vi "Init Airmar Serial.vi"(8 "error in (no error)":errorcluster, 10 "NotifierReff":T1, 11 "VISA Refnum in":refnum<visa-resource-name>="COM1") -> (0 "error out":errorcluster, 2 "Total number of connection attempts":i32, 3 "VISA Refnum out":refnum<visa-resource-name>)   [LabVIEW 2013]
doc: "This VI checks to see if the sensor is communicating on 4800 or 38400 baud and sets it to 38400 baud if it is not already."
uses:
  Data/TypeDefs/UTM Location.ctl
  Data/TypeDefs/Sail Set Suggestions.ctl
  Data/TypeDefs/Rudder Set Suggestions.ctl
  Data/TypeDefs/Notifiers.ctl
  Data/TypeDefs/OverrideMode.ctl
  Data/TypeDefs/OverrideInformation.ctl
  Data/TypeDefs/DynamixelSetupInfo.ctl
  Data/TypeDefs/MotorSetup.ctl
  Data/TypeDefs/AirmarStatus.ctl
panel:
  out "# of 38400 baud attempts":i32
  out "# of 4800 baud attempts":i32
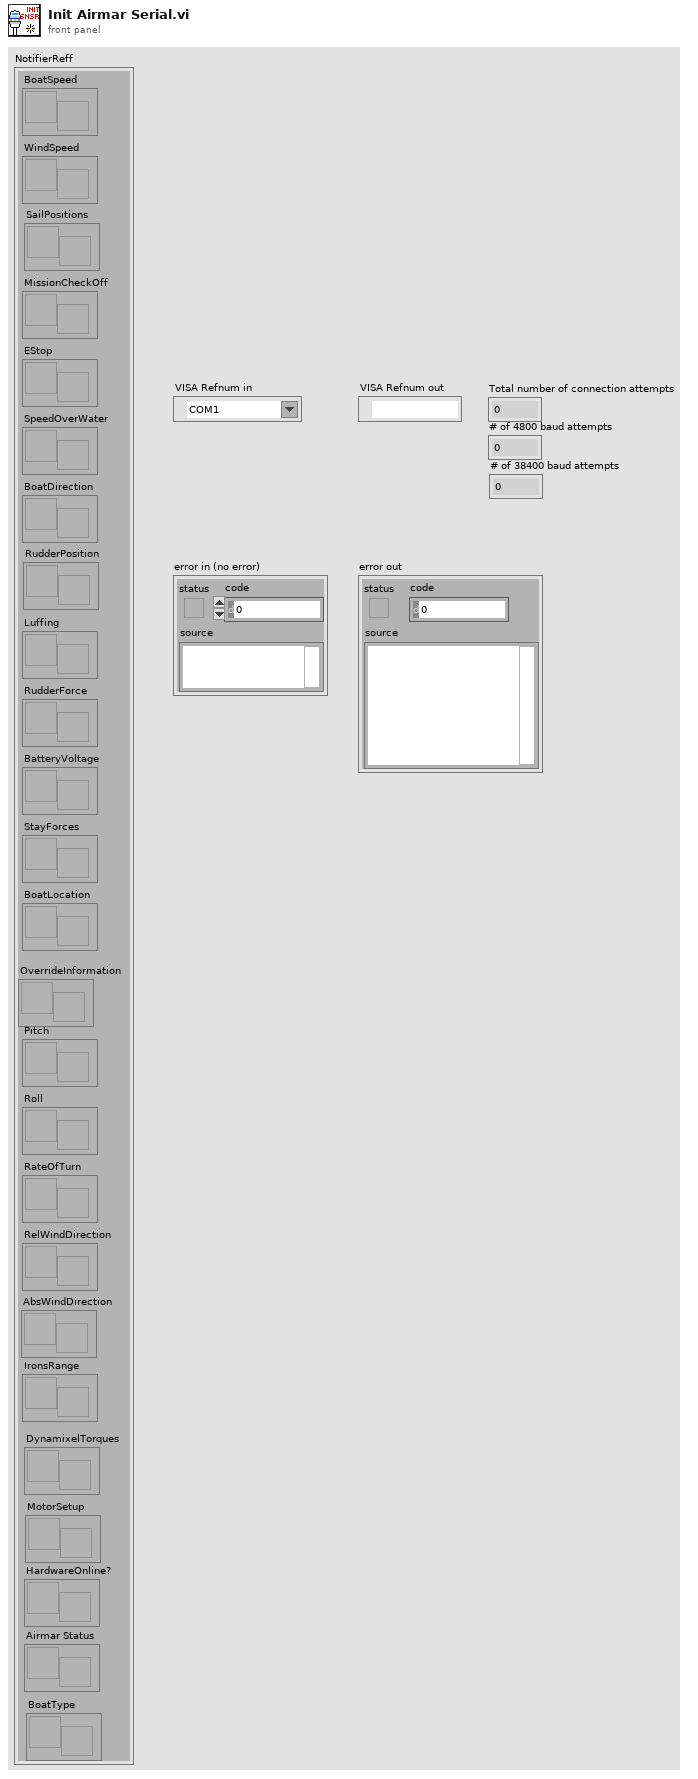
[diagram p1: front panel]
types:
  T1 = typedef "Notifiers.ctl" = cluster{"BoatSpeed":refnum<notifier>, "WindSpeed":refnum<notifier>, "MissionCheckOff":refnum<notifier>, "EStop":refnum<notifier>, "SpeedOverWater":refnum<notifier>, "BoatDirection":refnum<notifier>, "Luffing":refnum<notifier>, "RudderForce":refnum<notifier>, "BatteryVoltage":refnum<notifier>, "StayForces":refnum<notifier>, "BoatLocation":refnum<notifier>, "Pitch":refnum<notifier>, "Roll":refnum<notifier>, "RateOfTurn":refnum<notifier>, "RelWindDirection":refnum<notifier>, "SailPositions":refnum<notifier>, "RudderPosition":refnum<notifier>, "IronsRange":refnum<notifier>, "AbsWindDirection":refnum<notifier>, "OverrideInformation":refnum<notifier>, "DynamixelTorques":refnum<notifier>, "HardwareOnline?":refnum<notifier>, "MotorSetup":refnum<notifier>, "Airmar Status":refnum<notifier>, "BoatType":refnum<notifier>}
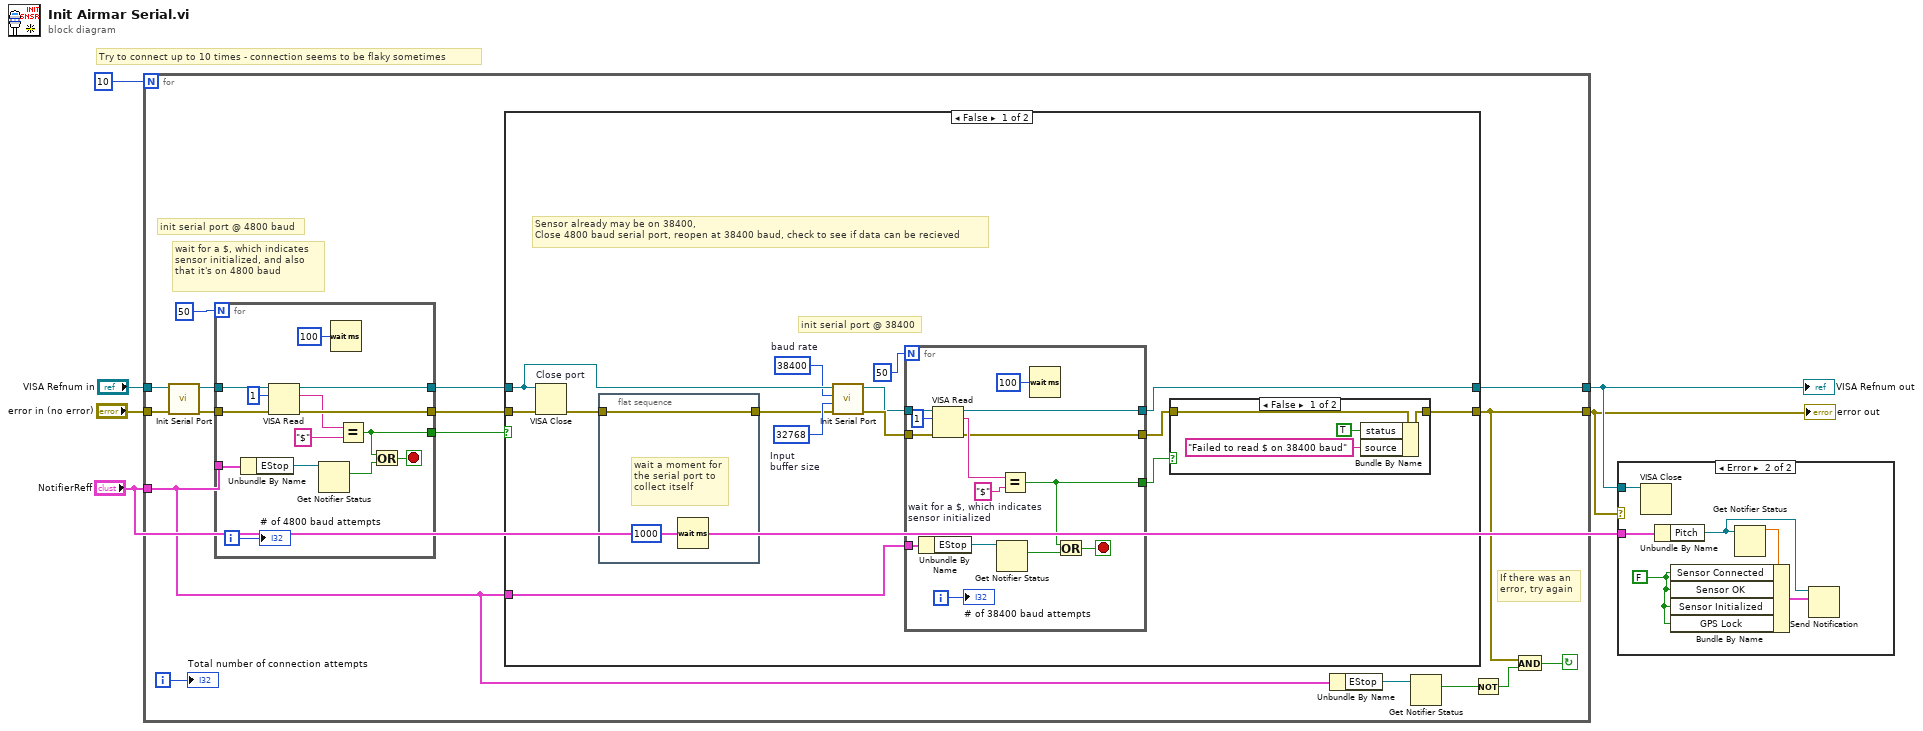
[diagram p0: block diagram]
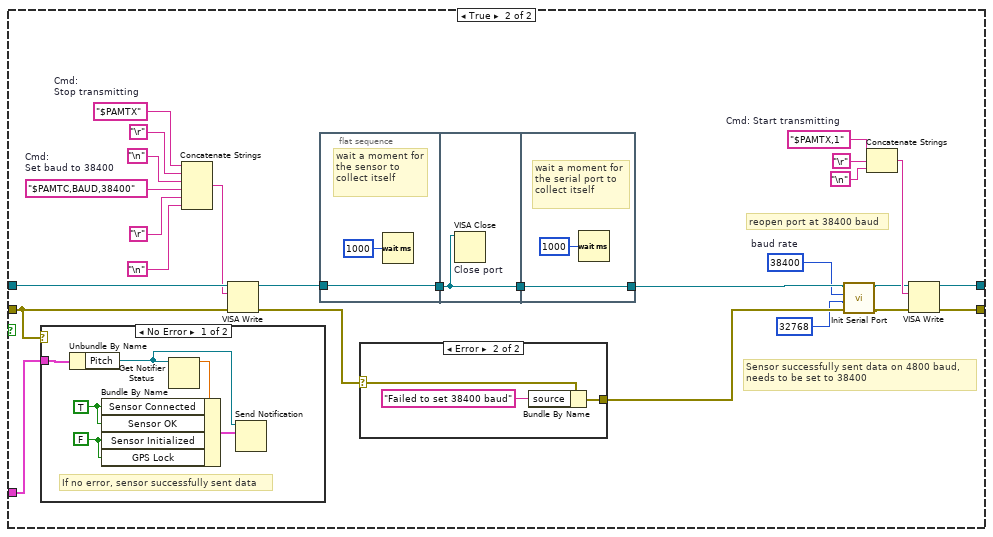
[diagram p3: hidden frame]
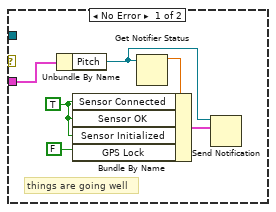
[diagram p6: hidden frame]
diagram:
  # "Try to connect up to 10 times - connection seems to be flaky sometimes"
  n1 = for {
    N: 10 -> [_]
    tunnel: "error in (no error)" -> [w12]
    tunnel: "VISA Refnum in" -> [w13]
    tunnel: [w22] -> w4
    tunnel: [w16] -> w3
    tunnel: "NotifierReff" -> [w8]
    i -> [w18]
    stop <- w17 continue-if-true
    # "If there was an \nerror, try again"
    # "wait for a $, which indicates sensor initialized, and also that it's on 4800 baud"
    # "init serial port @ 4800 baud"
    n2 = call "Init Serial Port.vi"("error in (no error)"=w12, "VISA Refnum in"=w13) -> ("error out"=w11:errorcluster, "VISA Refnum out"=w10:refnum<visa-resource-name>)  [unwired: 8 in]
    n3 = for {
      N: 50 -> [_]
      tunnel: [w36] -> w21
      tunnel: w10 -> [w35]
      tunnel: w11 -> [w34]
      tunnel: [w33] -> w20
      tunnel: [w28] -> w19
      tunnel: w8 -> [w26]
      i -> [w27]
      stop <- w29 stop-if-true
      n4 = Unbundle By Name(w26) -> ("EStop"=w25:refnum<notifier>)
      n5 = VISA Read(VISA resource name=w35, byte count=u32 1, error in (no error)=w34) -> (VISA resource name out=w36:refnum<visa-resource-name>, read buffer=w31:string, error out=w33:errorcluster)  [unwired: 1 out]
      n6 = Get Notifier Status(notifier=w25) -> (current notification=w24:bool)  [unwired: 1 in, 4 out]
      n7 = Wait (ms)(milliseconds to wait=u32 100) -> ()  [unwired: 1 out]
      n8 = Equal? ("wait for a $, which indicates\nsensor initialized")(x=w31, y="$" ("x")) -> (x = y?=w28:bool)
      n9 = Or(x=w28, y=w24) -> (x .or. y?=w29:bool)
      "# of 4800 baud attempts" <- w27
    }
    n10 = case shown="False" w19 {
      tunnel: [w50 w95] -> w22
      tunnel: w21 -> [w43 w90]
      tunnel: w20 -> [w45 w80]
      tunnel: [w49 w85] -> w16
      tunnel: w8 -> [w37 w72]
      frame False {
        w41 = u32 32768  # Input buffer size
        w42 = u32 38400  # baud rate
        # "init serial port @ 38400"
        # "Sensor already may be on 38400,\nClose 4800 baud serial port, reopen at 38400 baud, check to see if data can be recieved"
        n11 = VISA Close "Close port"(VISA resource name=w43, error in (no error)=w45) -> (error out=w44:errorcluster)
        n12 = flat-sequence {
          tunnel: w44 -> [w51]
          tunnel: [w51] -> w40
          frame #0 {
            # "wait a moment for the serial port to collect itself"
            n13 = Wait (ms)(milliseconds to wait=u32 1000) -> ()  [unwired: 1 out]
          }
        }
        n14 = call "Init Serial Port.vi"("error in (no error)"=w40, "Input\nbuffer size"=w41, "baud rate"=w42, "VISA Refnum in"=w43) -> ("error out"=w39:errorcluster, "VISA Refnum out"=w38:refnum<visa-resource-name>)  [unwired: 6 in]
        n15 = for {
          N: 50 -> [_]
          tunnel: w38 -> [w66]
          tunnel: w39 -> [w65]
          tunnel: [w64] -> w50
          tunnel: [w58] -> w48
          tunnel: [w60] -> w47
          tunnel: w37 -> [w55]
          i -> [w57]
          stop <- w59 stop-if-true
          n16 = Unbundle By Name(w55) -> ("EStop"=w56:refnum<notifier>)
          n17 = VISA Read(VISA resource name=w66, byte count=u32 1, error in (no error)=w65) -> (VISA resource name out=w64:refnum<visa-resource-name>, read buffer=w62:string, error out=w60:errorcluster)  [unwired: 1 out]
          n18 = Get Notifier Status(notifier=w56) -> (current notification=w53:bool)  [unwired: 1 in, 4 out]
          n19 = Equal? "wait for a $, which indicates\nsensor initialized"(x=w62, y="$" ("x")) -> (x = y?=w58:bool)
          n20 = Wait (ms)(milliseconds to wait=u32 100) -> ()  [unwired: 1 out]
          n21 = Or(x=w58, y=w53) -> (x .or. y?=w59:bool)
          "# of 38400 baud attempts" <- w57
        }
        n22 = case shown="False" w48 {
          tunnel: w47 -> [w68 w71]
          tunnel: [w67 w71] -> w49
          frame False {
            n23 = Bundle By Name(cluster=w68, "status"=TRUE, "source"="Failed to read $ on 38400 baud") -> (w67:errorcluster)
          }
          frame True {
          }
        }
      }
      frame True {
        w84 = "$PAMTC,BAUD,38400"  # Cmd: Set baud to 38400
        w89 = "$PAMTX"  # Cmd: Stop transmitting
        w94 = "$PAMTX,1"  # Cmd: Start transmitting
        w73 = u32 38400  # baud rate
        # "Sensor successfully sent data on 4800 baud,\nneeds to be set to 38400"
        # "reopen port at 38400 baud"
        n24 = case shown="No Error" w80 {
          tunnel: w72 -> [w107 _]
          frame No Error {
            w104 = FALSE
            w105 = TRUE
            # "If no error, sensor successfully sent data"
            n25 = Unbundle By Name(w107) -> ("Pitch"=w102:refnum<notifier>)
            n26 = Get Notifier Status(notifier=w102) -> (current notification=w106:dbl)  [unwired: 1 in, 4 out]
            n27 = Bundle By Name(cluster=w106, "Sensor Connected"=w105, "Sensor OK"=w105, "Sensor Initialized"=w104, "GPS Lock"=w104) -> (w103:cluster{})
            n28 = Send Notification(notification=w103, notifier=w102) -> ()  [unwired: 1 in, 2 out]
          }
          frame Error {
          }
        }
        n29 = Concatenate Strings(w89, "\r" ("Carriage Return Constant"), "\n", w84, "\r" ("Carriage Return Constant"), "\n") -> (w88:string)
        n30 = VISA Write(VISA resource name=w90, write buffer=w88, error in (no error)=w80) -> (VISA resource name out=w81:refnum<visa-resource-name>, error out=w79:errorcluster)  [unwired: 1 out]
        n31 = flat-sequence {
          tunnel: w81 -> [w108]
          tunnel: [w108] -> w97
          tunnel: w97 -> [w110]
          tunnel: [w110] -> w96
          tunnel: [w112] -> w78
          tunnel: w96 -> [w112]
          frame #0 {
            # "wait a moment for the sensor to collect itself"
            n32 = Wait (ms)(milliseconds to wait=u32 1000) -> ()  [unwired: 1 out]
          }
          frame #1 {
            n33 = VISA Close "Close port"(VISA resource name=w110) -> ()  [unwired: 1 in, 1 out]
          }
          frame #2 {
            # "wait a moment for the serial port to collect itself"
            n34 = Wait (ms)(milliseconds to wait=u32 1000) -> ()  [unwired: 1 out]
          }
        }
        n35 = case shown="Error" w79 {
          selector: w79 -> [w98 w101]
          tunnel: [w98 w99] -> w75
          frame No Error {
          }
          frame Error {
            n36 = Bundle By Name(cluster=w101, "source"="Failed to set 38400 baud") -> (w99:errorcluster)
          }
        }
        n37 = call "Init Serial Port.vi"("error in (no error)"=w75, "Input\nbuffer size"=u32 32768 ("Input\nbuffer size"), "baud rate"=w73, "VISA Refnum in"=w78) -> ("error out"=w76:errorcluster, "VISA Refnum out"=w77:refnum<visa-resource-name>)  [unwired: 6 in]
        n38 = Concatenate Strings(w94, "\r" ("Carriage Return Constant"), "\n") -> (w91:string)
        n39 = VISA Write(VISA resource name=w77, write buffer=w91, error in (no error)=w76) -> (VISA resource name out=w95:refnum<visa-resource-name>, error out=w85:errorcluster)  [unwired: 1 out]
      }
    }
    n40 = Unbundle By Name(w8) -> ("EStop"=w7:refnum<notifier>)
    n41 = Get Notifier Status(notifier=w7) -> (current notification=w9:bool)  [unwired: 1 in, 4 out]
    n42 = Not(x=w9) -> (.not. x?=w15:bool)
    n43 = And(x=w16, y=w15) -> (x .and. y?=w17:bool)
    "Total number of connection attempts" <- w18
  }
  "VISA Refnum out" <- w4
  "error out" <- w3
  n44 = case shown="Error" w3 {
    tunnel: w4 -> [_ w124]
    tunnel: "NotifierReff" -> [w113 w122]
    frame No Error {
      w114 = TRUE ("Sensor Connected")
      # "things are going well"
      n45 = Unbundle By Name(w113) -> ("Pitch"=w115:refnum<notifier>)
      n46 = Get Notifier Status(notifier=w115) -> (current notification=w117:dbl)  [unwired: 1 in, 4 out]
      n47 = Bundle By Name(cluster=w117, "Sensor Connected"=w114, "Sensor OK"=w114, "Sensor Initialized"=w114, "GPS Lock"=FALSE ("Sensor Connected")) -> (w116:cluster{})
      n48 = Send Notification(notification=w116, notifier=w115) -> ()  [unwired: 1 in, 2 out]
    }
    frame Error {
      w119 = FALSE
      n49 = VISA Close(VISA resource name=w124) -> ()  [unwired: 1 in, 1 out]
      n50 = Unbundle By Name(w122) -> ("Pitch"=w120:refnum<notifier>)
      n51 = Get Notifier Status(notifier=w120) -> (current notification=w123:dbl)  [unwired: 1 in, 4 out]
      n52 = Bundle By Name(cluster=w123, "Sensor Connected"=w119, "Sensor OK"=w119, "Sensor Initialized"=w119, "GPS Lock"=w119) -> (w121:cluster{})
      n53 = Send Notification(notification=w121, notifier=w120) -> ()  [unwired: 1 in, 2 out]
    }
  }
